vi "Launch.vi"(8 "error in (no error)":errorcluster, 11 "Response Channel":refnum<class "Messenger.lvclass">) -> (0 "error out":errorcluster, 3 "Actor API out":refnum<class "Actor API.lvclass">)   [LabVIEW 2015, in "Debugger.lvclass"]
doc: "<b>Response</b> channel is used by this actor to return infomation back to the parent. Typically this input is the Request channel of the parent actor."
uses:
  Debugger.lvclass
  Base Actor/API/Actor API.lvclass
  Messaging/Messenger/Messenger.lvclass
  Base Actor/Actor/Front Panel State.ctl
  Base Actor/Actor/Actor.lvclass
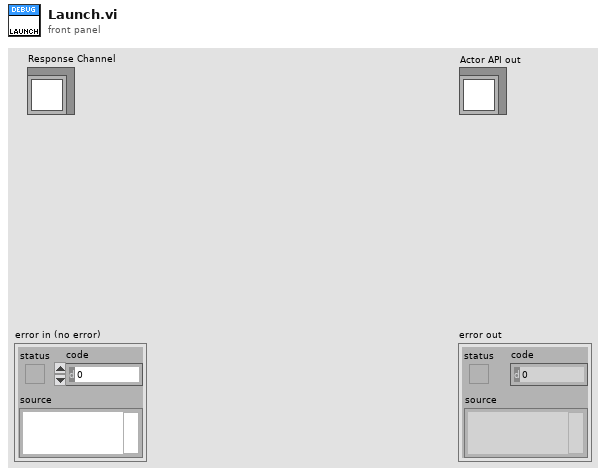
[diagram p1: front panel]
types:
  T1 = typedef "Actor.lvclass/Front Panel State.ctl" = enum32{"Invalid", "Standard", "Closed", "Hidden", "Minimized", "Maximized"}
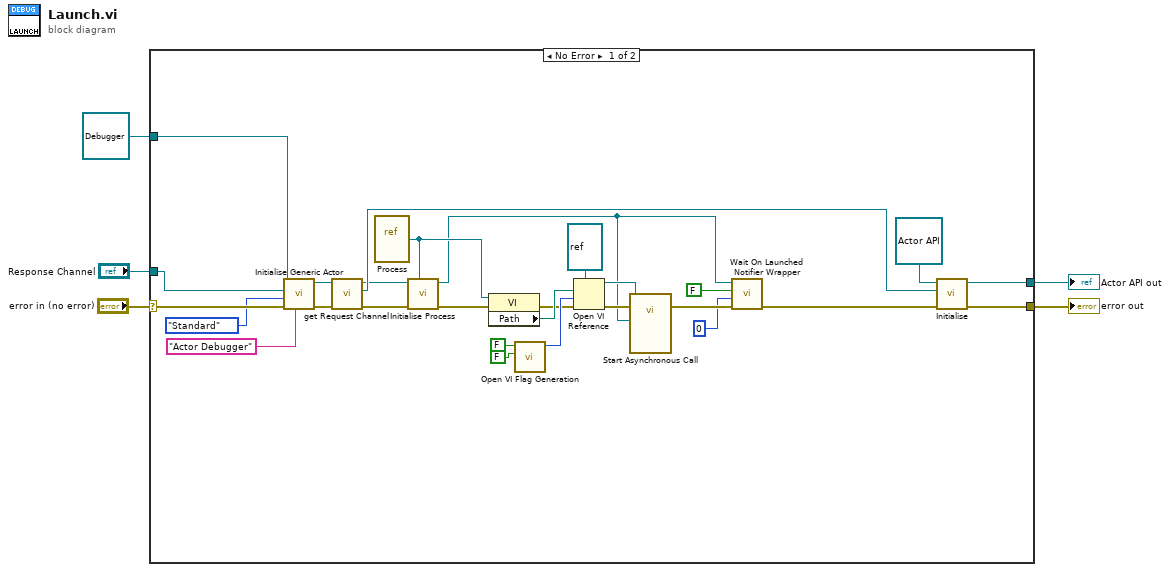
[diagram p0: block diagram]
diagram:
  n1 = case shown="No Error" "error in (no error)" {
    selector: "error in (no error)" -> [w24 w33]
    tunnel: [w19 w33] -> w5
    tunnel: [w11 _] -> w2
    tunnel: refnum<class "Debugger.lvclass"> refnum ("Worker Test 1.lvclass") -> [w22 _]
    tunnel: "Response Channel" -> [w8 _]
    frame No Error {
      n2 = call-dynamic "Initialise Generic Actor.vi"("Name"="Actor Debugger", "Front Panel State"=Front_Panel_State."Standard", "Response Channel"=w8, "Actor in"=w22) -> ("Actor out"=w25:refnum<class "Debugger.lvclass">)  [unwired: 6 in, 1 out]
      n3 = call "get Request Channel.vi"("error in (no error)"=w24, "Actor in"=w25) -> ("error out"=w15:errorcluster, "Request Channel"=w26:refnum<class "Messenger.lvclass">, "Actor out"=w14:refnum<class "Debugger.lvclass">)  [unwired: 7 in]
      n4 = vi-ref "Process.vi"() -> (w12:refnum<vi>)
      n5 = call-dynamic "Initialise Process.vi"("Process"=w12, "error in (no error)"=w15, "Actor in"=w14) -> ("error out"=w13:errorcluster, "Actor out"=w7:refnum<class "Debugger.lvclass">)  [unwired: 7 in]
      n6 = property class="VI"(reference=w12, error in=w13) -> (error out=w17:errorcluster, "Path"=w18:path)  [unwired: 1 out]
      n7 = call "Open VI Flag Generation.vi"("Call And Collect (F)"=FALSE, "Re-entrant (F)"=FALSE) -> ("Flags"=w32:i32)  [unwired: 9 in]
      n8 = Open VI Reference(type specifier VI Refnum (for type only)=refnum<vi> refnum, vi path=w18, options=w32, error in (no error)=w17) -> (vi reference=w28:refnum<vi>, error out=w27:errorcluster)  [unwired: 2 in]
      n9 = call-by-ref "Start Asynchronous Call"(reference=w28, error in=w27, "Worker Test 1.lvclass"=w7) -> (error out=w23:errorcluster)  [unwired: 11 in, 1 out]
      n10 = call-dynamic "Wait On Launched Notifier Wrapper.vi"("error in (no error)"=w23, "Launch Timeout [ms]"=0, "Wait For Launch Completed"=FALSE ("Wait For Launch Completed (F)"), "Actor in"=w7) -> ("error out"=w6:errorcluster)  [unwired: 5 in, 2 out]
      n11 = call "Initialise.vi"("error in (no error)"=w6, "Request Channel"=w26, "Actor API in"=refnum<class "Actor API.lvclass"> refnum ("Actor API.lvclass")) -> ("error out"=w19:errorcluster, "Actor API out"=w11:refnum<class "Actor API.lvclass">)  [unwired: 7 in]
    }
    frame Error {
    }
  }
  "error out" <- w5
  "Actor API out" <- w2
